vi "Ideal Result.vi"(8 "Error in":errorcluster, 11 "DAC in":refnum<class "DAC.lvclass">) -> (0 "Error out":errorcluster, 3 "DAC out":refnum<class "DAC.lvclass">)   [LabVIEW 2020, in "DAC.lvclass"]
doc: "Geneartes Ideal value for DAC"
uses:
  DAC.lvclass
  D:/SDLC/Class/INL DNL Test/Device/Parent/Device.lvclass
  DAC.lvclass/DAC.ctl
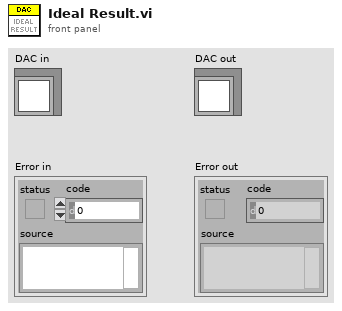
[diagram p1: front panel]
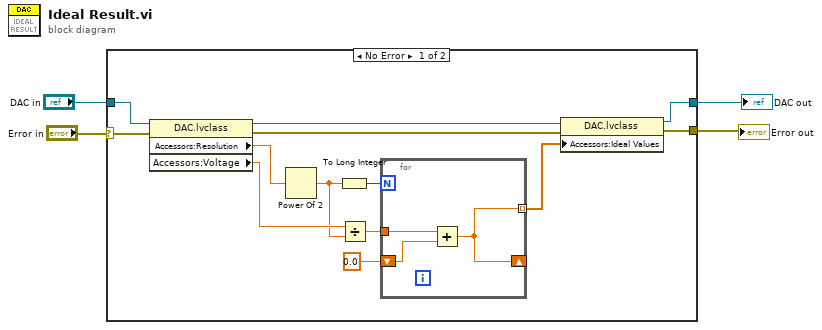
[diagram p0: block diagram]
diagram:
  n1 = case shown="No Error" "Error in" {
    selector: "Error in" -> [w16 w21]
    tunnel: "DAC in" -> [w17 w22]
    tunnel: [w9 w22] -> w2
    tunnel: [w8 w21] -> w1
    frame No Error {
      n2 = property class="DAC.lvclass"(reference=w17, error in=w16) -> (reference out=w12:refnum<class "DAC.lvclass">, error out=w11:errorcluster, "Accessors:Resolution"=w15:dbl, "Accessors:Voltage"=w7:dbl)
      n3 = Power Of 2(x=w15) -> (2^x=w6:dbl)
      n4 = To Long Integer(number=w6) -> (32bit integer=w14:i32)
      n5 = Divide(x=w7, y=w6) -> (x/y=w5:dbl)
      n6 = for {
        N: w14 -> [_]
        shift-right: [w19] -> _
        shift-left: 0.0 -> [w20]
        tunnel: [w19] -> w10 mode=indexing
        tunnel: w5 -> [w18]
        n7 = Add(x=w18, y=w20) -> (x+y=w19:dbl)
      }
      n8 = property class="DAC.lvclass"(reference=w12, error in=w11, "Accessors:Ideal Values"=w10) -> (reference out=w9:refnum<class "DAC.lvclass">, error out=w8:errorcluster)
    }
    frame Error {
    }
  }
  "Error out" <- w1
  "DAC out" <- w2
